vi "arduino_4_0.vi"() -> ()   [LabVIEW 2015]
uses:
  <vilib>/LabVIEW Interface for Arduino/LabVIEW Interface for Arduino.lvlib
panel:
  in  "stop":bool
  in  "PWM Pin (3)":u8=3
  in  "Control Led intensity":dbl(knob) scale=0.0..255.0
  in  "VISA resource":refnum<visa-resource-name>
  # "LED connect arduino pin 3 pwm when you change the knobe value led intensity change"
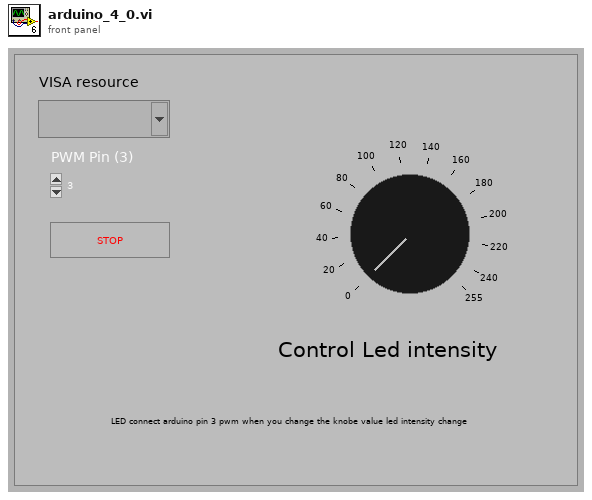
[diagram p1: front panel]
types:
  T1 = typedef "LabVIEW Interface for Arduino.lvlib/Arduino Resource.ctl" = cluster{"VISA resource":refnum<visa-resource-name>, "Board Type":T2, "Connection Type":enum8{"USB / Serial"}, "Bytes Per Packet (15)":u8}
  T2 = typedef "LabVIEW Interface for Arduino.lvlib/Board Type.ctl" = enum16{"Uno", "Dimuelanove w/Atmega 328", "Mega 2560"}
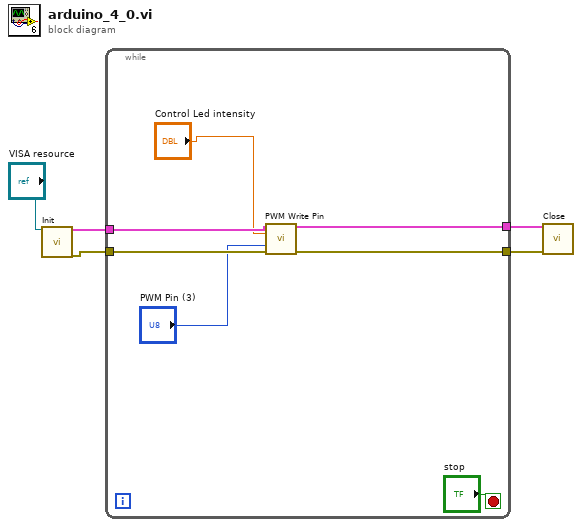
[diagram p0: block diagram]
diagram:
  n1 = call <vilib>:"Init.vi"("VISA resource"="VISA resource") -> ("Arduino Resource"=w5:T1, "error out"=w3:errorcluster)  [unwired: 17 in]
  n2 = while {
    tunnel: w5 -> [w12]
    tunnel: [w11] -> w4
    tunnel: w3 -> [w10]
    tunnel: [w9] -> w2
    stop <- "stop" stop-if-true
    n3 = call <vilib>:"PWM Write Pin.vi"("Arduino Resource"=w12, "Duty Cycle (0 - 255)"="Control Led intensity", "PWM Pin (3)"="PWM Pin (3)", "error in"=w10) -> ("Arduino Resource"=w11:T1, "error out"=w9:errorcluster)  [unwired: 10 in]
  }
  n4 = call <vilib>:"Close.vi"("Arduino Resource"=w4, "error in"=w2) -> ()  [unwired: 13 in, 1 out]
